vi "TREE_List Symbol Custom.vi"(8 "error in":errorcluster, 9 "PicturePath":path, 10 "Tags":string[](array[string]), 11 "ListRef":refnum<vi>) -> (0 "error out":errorcluster, 3 "ListRef Out":refnum<vi>)   [LabVIEW 2016]
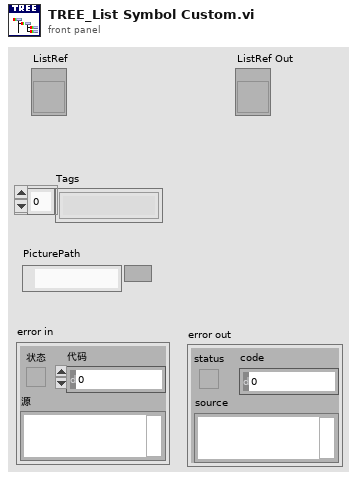
[diagram p1: front panel]
types:
  T1 = enum32{"invalid app kind", "Development System", "Run Time System", "Student Edition", "Embedded LabVIEW", "Evaluation", "Custom"}
  T2 = typedef "imagedata.ctl" = cluster{"image type":i32, "image depth":i32, "image":u8[], "mask":u8[], "colors":u32[], "Rectangle":cluster{"left":i16, "top":i16, "right":i16, "bottom":i16}}
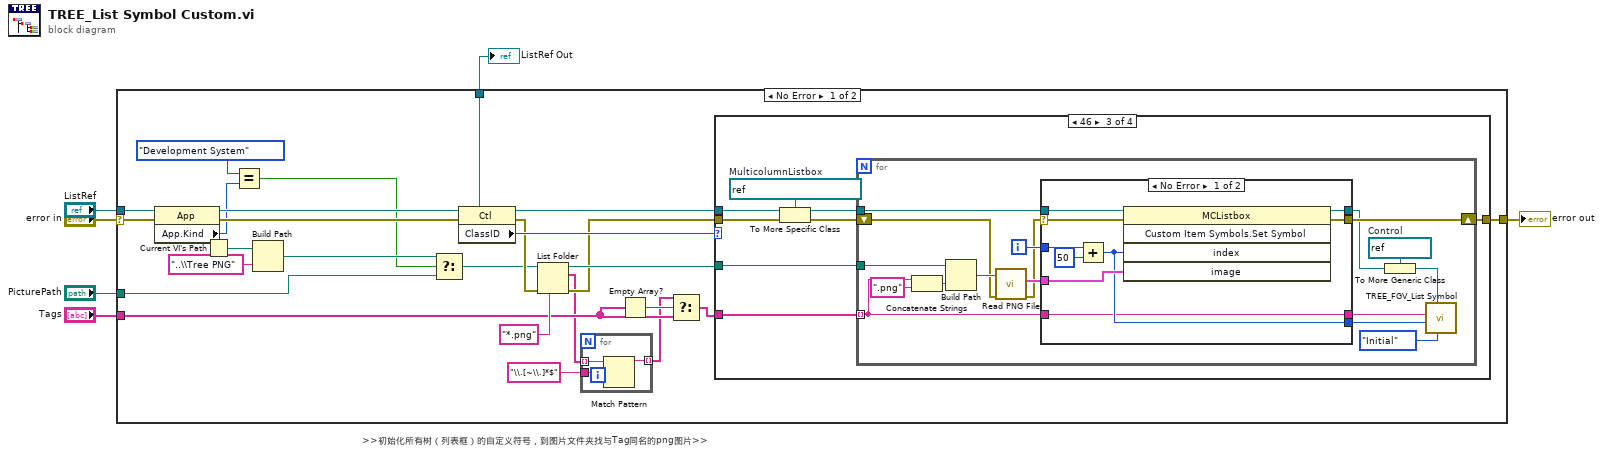
[diagram p0: block diagram]
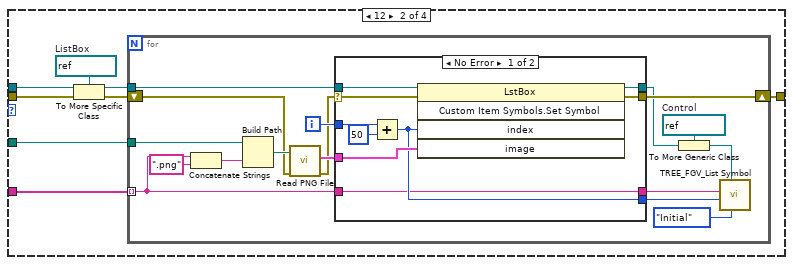
[diagram p3: hidden frame]
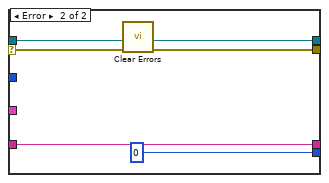
[diagram p4: hidden frame]
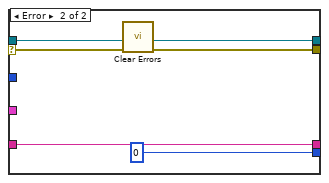
[diagram p5: hidden frame]
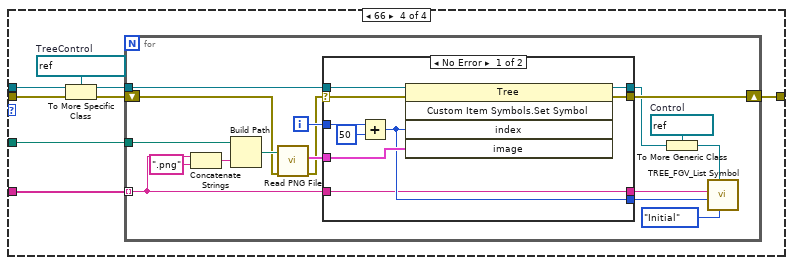
[diagram p6: hidden frame]
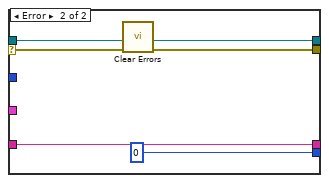
[diagram p7: hidden frame]
diagram:
  # ">>初始化所有树（列表框）的自定义符号，到图片文件夹找与Tag同名的png图片>>"
  n1 = case shown="No Error" "error in" {
    selector: "error in" -> [w12 w152]
    tunnel: [w30 w152] -> w6
    tunnel: "ListRef" -> [w29 w153]
    tunnel: [w28 w153] -> w4
    tunnel: "Tags" -> [w25 _]
    tunnel: "PicturePath" -> [w7 _]
    frame No Error {
      n2 = property class="App"(error in=w12) -> (error out=w11:errorcluster, "App.Kind"=w10:T1)  [unwired: 1 in, 1 out]
      n3 = Current VI's Path() -> (path=w15:path)
      n4 = Equal?(x=T1."Development System", y=w10) -> (x = y?=w8:bool)
      n5 = Build Path(base path=w15, name or relative path="..\\Tree PNG" ("名称或相对路径")) -> (appended path=w14:path)
      n6 = Select(t=w14, s=w8, f=w7) -> (s? t:f=w16:path)
      n7 = property class="Ctl"(reference=w29, error in=w11) -> (reference out=w28:refnum<vi>, error out=w22:errorcluster, "ClassID"=w27:u32)
      n8 = List Folder(path=w16, pattern="*.png" ("string"), error in=w22) -> (path out=w23:path, filenames=w18:string[], error out=w21:errorcluster)  [unwired: 1 in, 1 out]
      n9 = for {
        tunnel: "\\.[~\\.]*$" ("regular expression") -> [w33]
        tunnel: w18 -> [w32] mode=indexing
        tunnel: [w31] -> w17 mode=indexing
        n10 = Match Pattern(string=w32, regular expression=w33) -> (before substring=w31:string)  [unwired: 4 out]
      }
      n11 = Empty Array?(array=w25) -> (empty?=w20:bool)
      n12 = Select(t=w17, s=w20, f=w25) -> (s? t:f=w24:string[])
      n13 = case shown="46" w27 {
        tunnel: w23 -> [_ w42 w81 w113]
        tunnel: w24 -> [_ w41 w80 w114]
        tunnel: [w34 w40 w79 w120] -> w30
        tunnel: w28 -> [_ w39 w78 w119]
        tunnel: w21 -> [w34 w36 w75 w116]
        frame 0, Default {
        }
        frame 12 {
          w37 = refnum<vi> refnum  # ListBox
          n14 = To More Specific Class(target class=w37, reference=w39, error in=w36) -> (specific class reference=w38:refnum<vi>, error out=w35:errorcluster)
          n15 = for {
            tunnel: w42 -> [w59]
            shift-right: [w54] -> w40
            shift-left: w35 -> [w57]
            tunnel: w41 -> [w44] mode=indexing
            tunnel: w38 -> [w52]
            i -> [w55]
            w48 = refnum<vi> refnum  # Control
            n16 = Concatenate Strings(w44, ".png" ("string")) -> (w43:string)
            n17 = Build Path(base path=w59, name or relative path=w43) -> (appended path=w58:path)
            n18 = call <vilib>:"Read PNG File.vi"("error in (no error)"=w57, "path to PNG file"=w58) -> ("error out"=w51:errorcluster, "image data"=w56:T2)  [unwired: 7 in, 1 out]
            n19 = case shown="No Error" w51 {
              selector: w51 -> [w62 w72]
              tunnel: w56 -> [w68 _]
              tunnel: w55 -> [w67 _]
              tunnel: [w65 w71] -> w54
              tunnel: [w64 w73] -> w47
              tunnel: w52 -> [w63 w73]
              tunnel: w44 -> [w60 w70]
              tunnel: [w60 w70] -> w50
              tunnel: [w61 0] -> w49
              frame No Error {
                n20 = Add(x=w67, y=50) -> (x+y=w61:i32)
                n21 = invoke class="LstBox" method="Custom Item Symbols.Set Symbol"(reference=w63, error in=w62, "index"=w61, "image"=w68) -> (reference out=w64:refnum<vi>, error out=w65:errorcluster)  [unwired: 1 in, 3 out]
              }
              frame Error {
                n22 = call <vilib>:"Clear Errors.vi"("error in (no error)"=w72) -> ("error out"=w71:errorcluster)  [unwired: 5 in, 1 out]
              }
            }
            n23 = To More Generic Class(target class=w48, reference=w47) -> (generic class reference=w46:refnum<vi>)
            n24 = call "TREE_FGV_List Symbol.vi"("Oper"=enum16{"Initial", "Get Symbol", "Clear"}."Initial", "Control"=w46, "Symbol"=w49, "Picture Name"=w50) -> ()  [unwired: 7 in, 1 out]
          }
        }
        frame 46 {
          w76 = refnum<vi> refnum  # MulticolumnListbox
          n25 = To More Specific Class(target class=w76, reference=w78, error in=w75) -> (specific class reference=w77:refnum<vi>, error out=w74:errorcluster)
          n26 = for {
            tunnel: w81 -> [w98]
            shift-right: [w93] -> w79
            shift-left: w74 -> [w96]
            tunnel: w80 -> [w83] mode=indexing
            tunnel: w77 -> [w91]
            i -> [w94]
            w87 = refnum<vi> refnum  # Control
            n27 = Concatenate Strings(w83, ".png" ("string")) -> (w82:string)
            n28 = Build Path(base path=w98, name or relative path=w82) -> (appended path=w97:path)
            n29 = call <vilib>:"Read PNG File.vi"("error in (no error)"=w96, "path to PNG file"=w97) -> ("error out"=w90:errorcluster, "image data"=w95:T2)  [unwired: 7 in, 1 out]
            n30 = case shown="No Error" w90 {
              selector: w90 -> [w101 w111]
              tunnel: w95 -> [w107 _]
              tunnel: w94 -> [w106 _]
              tunnel: [w104 w110] -> w93
              tunnel: [w103 w112] -> w86
              tunnel: w91 -> [w102 w112]
              tunnel: w83 -> [w99 w109]
              tunnel: [w99 w109] -> w89
              tunnel: [w100 0] -> w88
              frame No Error {
                n31 = Add(x=w106, y=50) -> (x+y=w100:i32)
                n32 = invoke class="MCListbox" method="Custom Item Symbols.Set Symbol"(reference=w102, error in=w101, "index"=w100, "image"=w107) -> (reference out=w103:refnum<vi>, error out=w104:errorcluster)  [unwired: 1 in, 3 out]
              }
              frame Error {
                n33 = call <vilib>:"Clear Errors.vi"("error in (no error)"=w111) -> ("error out"=w110:errorcluster)  [unwired: 5 in, 1 out]
              }
            }
            n34 = To More Generic Class(target class=w87, reference=w86) -> (generic class reference=w85:refnum<vi>)
            n35 = call "TREE_FGV_List Symbol.vi"("Oper"=enum16{"Initial", "Get Symbol", "Clear"}."Initial", "Control"=w85, "Symbol"=w88, "Picture Name"=w89) -> ()  [unwired: 7 in, 1 out]
          }
        }
        frame 66 {
          w117 = refnum<vi> refnum  # TreeControl
          n36 = To More Specific Class(target class=w117, reference=w119, error in=w116) -> (specific class reference=w118:refnum<vi>, error out=w115:errorcluster)
          n37 = for {
            tunnel: w113 -> [w137]
            shift-right: [w132] -> w120
            shift-left: w115 -> [w135]
            tunnel: w114 -> [w122] mode=indexing
            tunnel: w118 -> [w130]
            i -> [w133]
            w126 = refnum<vi> refnum  # Control
            n38 = Concatenate Strings(w122, ".png" ("string")) -> (w121:string)
            n39 = Build Path(base path=w137, name or relative path=w121) -> (appended path=w136:path)
            n40 = call <vilib>:"Read PNG File.vi"("error in (no error)"=w135, "path to PNG file"=w136) -> ("error out"=w129:errorcluster, "image data"=w134:T2)  [unwired: 7 in, 1 out]
            n41 = case shown="No Error" w129 {
              selector: w129 -> [w140 w150]
              tunnel: w134 -> [w146 _]
              tunnel: w133 -> [w145 _]
              tunnel: [w143 w149] -> w132
              tunnel: [w142 w151] -> w125
              tunnel: w130 -> [w141 w151]
              tunnel: w122 -> [w138 w148]
              tunnel: [w138 w148] -> w128
              tunnel: [w139 0] -> w127
              frame No Error {
                n42 = Add(x=w145, y=50) -> (x+y=w139:i32)
                n43 = invoke class="Tree" method="Custom Item Symbols.Set Symbol"(reference=w141, error in=w140, "index"=w139, "image"=w146) -> (reference out=w142:refnum<vi>, error out=w143:errorcluster)  [unwired: 1 in, 3 out]
              }
              frame Error {
                n44 = call <vilib>:"Clear Errors.vi"("error in (no error)"=w150) -> ("error out"=w149:errorcluster)  [unwired: 5 in, 1 out]
              }
            }
            n45 = To More Generic Class(target class=w126, reference=w125) -> (generic class reference=w124:refnum<vi>)
            n46 = call "TREE_FGV_List Symbol.vi"("Oper"=enum16{"Initial", "Get Symbol", "Clear"}."Initial", "Control"=w124, "Symbol"=w127, "Picture Name"=w128) -> ()  [unwired: 7 in, 1 out]
          }
        }
      }
    }
    frame Error {
    }
  }
  "error out" <- w6
  "ListRef Out" <- w4
